vi "set_DSC.vi"(0 "Host_Reference":refnum<class "HGF_Reference.lvclass">, 1 "DSCException":refnum<class "HGF_TriggeredEvent.lvclass">, 2 "Host_Event":refnum<class "HGF_Event.lvclass">, 3 "Agent_Event":refnum<class "HGF_Event.lvclass">, 4 "ManagerEvent":refnum<class "HGF_Event.lvclass">, 5 "error in (no error)":errorcluster, 6 "DSCDestination":refnum<class "HGF_TriggeredEvent.lvclass">, 7 "Host Variable":refnum<k21>, 8 "timeout in ms (-1)":i32=-1, 9 "MoAgSy_DSCThreadPool":refnum<class "HGF_Reference.lvclass">) -> (14 "dup Host_Reference":refnum<class "HGF_Reference.lvclass">, 19 "error out":errorcluster)   [LabVIEW 2009, in "MoAgSy.lvlib" / "MoAgSy_Host.lvclass"]
doc: "<B>public</B> VI sets DSC settings for referenced Host.\nThese are the DSC event based variable monitor, a variable manager to create and delete variables dynamically and the host variable.\nCalled during DSC init process.\n\nF.Berck@gsi.de\nGSI Darmstadt 2009"
uses:
  MoAgSy_Host.lvclass
  HGF_BaseClasses/HGF_Reference/HGF_Reference.lvclass
  HGF_BaseClasses/HGF_Event/HGF_Event.lvclass
  HGF_BaseClasses/HGF_TriggeredEvent/HGF_TriggeredEvent.lvclass
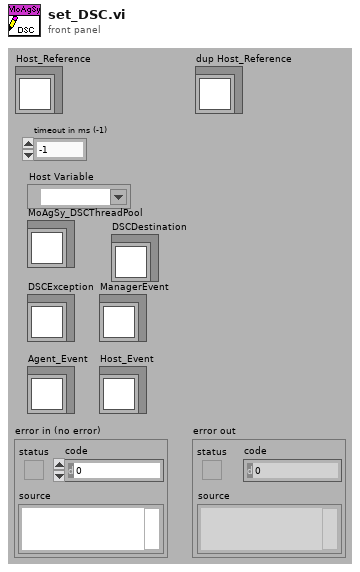
[diagram p1: front panel]
types:
  T1 = cluster{"Host Variable":refnum<k21>, "Agent_Event (Monitor Event)":refnum<class "HGF_Event.lvclass">, "Host_Event (Monitor Event)":refnum<class "HGF_Event.lvclass">, "DSCException":refnum<class "HGF_TriggeredEvent.lvclass">, "MoAgSy_DSCThreadPool":refnum<class "HGF_Reference.lvclass">, "ManagerEvent":refnum<class "HGF_Event.lvclass">, "DSCDestination":refnum<class "HGF_TriggeredEvent.lvclass">}
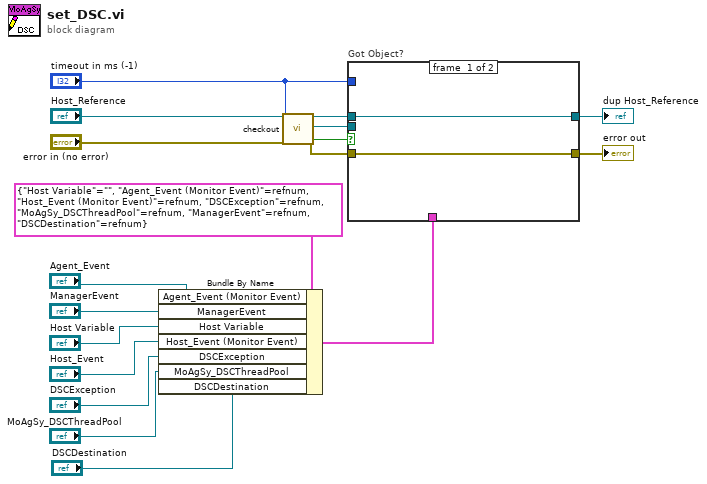
[diagram p0: block diagram]
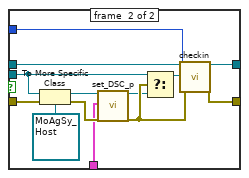
[diagram p2: hidden frame]
diagram:
  n1 = Bundle By Name(cluster=T1 {"Host Variable"="", "Agent_Event (Monitor Event)"=refnum, "Host_Event (Monitor Event)"=refnum, "DSCException"=refnum, "MoAgSy_DSCThreadPool"=refnum, "ManagerEvent"=refnum, "DSCDestination"=refnum} ("DSC"), "Agent_Event (Monitor Event)"="Agent_Event", "ManagerEvent"="ManagerEvent", "Host Variable"="Host Variable", "Host_Event (Monitor Event)"="Host_Event", "DSCException"="DSCException", "MoAgSy_DSCThreadPool"="MoAgSy_DSCThreadPool", "DSCDestination"="DSCDestination") -> (w9:T1)
  n2 = call "checkout.vi"("HGF_Reference"="Host_Reference", "timeout in ms (-1)"="timeout in ms (-1)", "error in (no error)"="error in (no error)") -> ("dup HGF_Reference"=w13:refnum<class "HGF_Reference.lvclass">, "Object"=w11:refnum<class>, "got object?"=w12:bool, "error out"=w10:errorcluster)  [unwired: 13 out]
  n3 = case "Got Object?" shown="True" w12 {
    tunnel: w11 -> [_ w25]
    tunnel: w13 -> [w20 w32]
    tunnel: [w20 w31] -> w17
    tunnel: "timeout in ms (-1)" -> [_ w30]
    tunnel: [w19 w29] -> w16
    tunnel: w10 -> [w19 w28]
    tunnel: w9 -> [_ w21]
    frame #0 {
    }
    frame #1 {
      n4 = To More Specific Class(target class=refnum<class "MoAgSy_Host.lvclass"> refnum ("MoAgSy.lvlib:MoAgSy_Host.lvclass"), reference=w25, error in=w28) -> (specific class reference=w27:refnum<class "MoAgSy_Host.lvclass">, error out=w26:errorcluster)
      n5 = call "set_DSC_p.vi"("MoAgSy_Host"=w27, "DSC"=w21, "error in (no error)"=w26) -> ("dup MoAgSy_Host"=w22:refnum<class "MoAgSy_Host.lvclass">, "error out"=w23:errorcluster)  [unwired: 15 out]
      n6 = Select(t=w25, s=w23, f=w22) -> (s? t:f=w24:refnum<class>)
      n7 = call "checkin.vi"("HGF_Reference"=w32, "Object"=w24, "timeout /ms (-1)"=w30, "error in (no error)"=w23) -> ("dup HGF_Reference"=w31:refnum<class "HGF_Reference.lvclass">, "error out"=w29:errorcluster)  [unwired: 14 out]
    }
  }
  "dup Host_Reference" <- w17
  "error out" <- w16
